vi "Parse GET Headers.vi"(11 "headers":string="HTTP/1.1 200 OK\r\nAccess-Control-Expose-Headers: Content-Length\r\nETag: \"v3a0\"\r\nExpires: Sat, 18 Jan 2020 16:15:15 GMT\r\nContent-Disposition: inline;filename=\"unnamed.jpg\"\r\nContent-Type: image/jpeg\r\nVary: Origin\r\nAccess-Control-Allow-Origin: *\r\nTiming-Allow-Origin: *\r\nX-Content-Type-Options: nosniff\r\nDate: Fri, 17 Jan 2020 20:37:42 GMT\r\nServer: fife\r\nContent-Length: 2537\r\nX-XSS-Protection: 0\r\nAge: 449\r\nCache-Control: public, max-age=86400, no-transform\r\nAlt-Svc: quic=\":443\"; ma=2592000; v=\"46,43\",h3-Q050=\":443\"; ma=2592000,h3-Q049=\":443\"; ma=2592000,h3-Q048=\":443\"; ma=2592000,h3-Q046=\":443\"; ma=2592000,h3-Q043=\":443\"; ma=2592000\r\n\r\n") -> (3 "map":map{string, string}(c390))   [LabVIEW 2020]
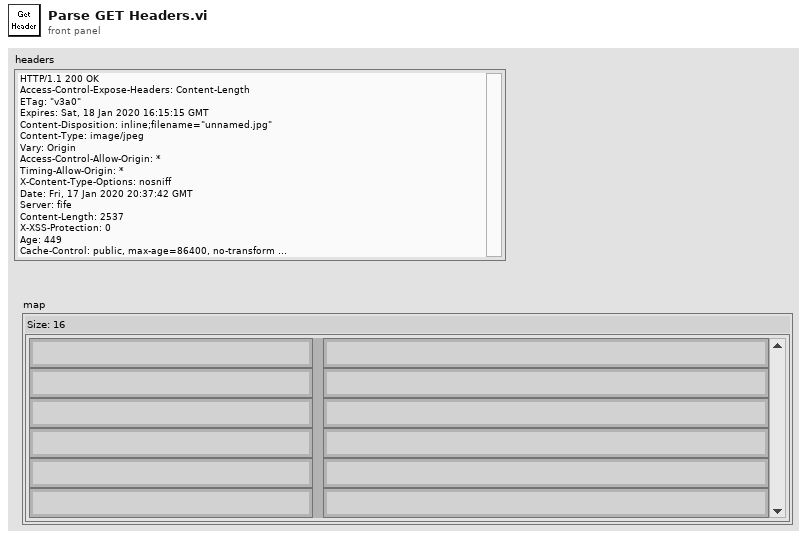
[diagram p1: front panel]
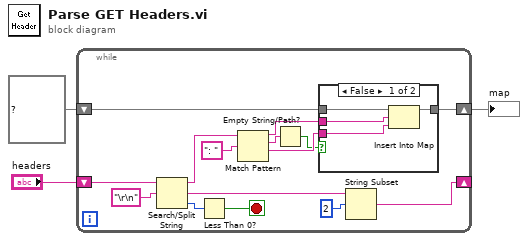
[diagram p0: block diagram]
diagram:
  n1 = while {
    shift-right: [w17] -> w2
    shift-left: map{string, string} {} ("map") -> [w18]
    shift-right: [w4] -> _
    shift-left: "headers" -> [w12]
    stop <- w16 stop-if-true
    n2 = Search/Split String(string=w12, search string/char (-)="\r\n") -> (substring before match=w10:string, match + rest of string=w6:string, offset of match=w7:i32)  [unwired: 1 in]
    n3 = Less Than 0?(x=w7) -> (x < 0?=w16:bool)
    n4 = Match Pattern(string=w10, regular expression=": ") -> (before substring=w14:string, match substring=w9:string, after substring=w13:string)  [unwired: 1 in, 1 out]
    n5 = Empty String/Path?(string/path=w9) -> (empty?=w8:bool)
    n6 = case shown="False" w8 {
      tunnel: w18 -> [w22 w23]
      tunnel: [w21 w23] -> w17
      tunnel: w14 -> [w20 _]
      tunnel: w13 -> [w19 _]
      frame False {
        n7 = Insert Into Map(map in=w22, key=w20, value=w19) -> (map out=w21:map{string, string})  [unwired: 2 out]
      }
      frame True {
      }
    }
    n8 = String Subset(string=w6, offset (0)=2) -> (substring=w4:string)  [unwired: 1 in]
  }
  "map" <- w2
